vi "Degrees to Position.vi"(4 "Degree":dbl) -> (1 "Encoder Position":dbl)   [LabVIEW 2019]
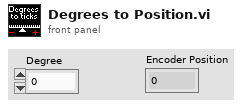
[diagram p1: front panel]
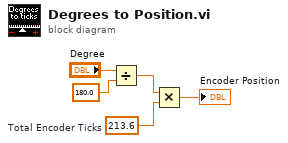
[diagram p0: block diagram]
diagram:
  w2 = 213.6  # Total Encoder Ticks
  n1 = Divide(x="Degree", y=180.0) -> (x/y=w3:dbl)
  n2 = Multiply(x=w3, y=w2) -> (x*y=→"Encoder Position":dbl)
